vi "Reset.vi"(8 "error in (no error)":errorcluster, 10 "gRPCid":T4, 11 "ctet_dmm":T1) -> (0 "error out":errorcluster, 3 "ctet_dmm out":T1)   [LabVIEW 2019, in "ctet_dmm User Library.lvlib"]
uses:
  ctet_dmm User Library.lvlib
  Servers/ctet_dmm/gRPC lvSupport/Server API/typeDefs/grpcId.ctl
  Types/ctet_dmm.ctl
  Servers/ctet_dmm/ctet_dmm Class/RPC Messages/measurementservice_DMMConfigResponse/measurementservice_DMMConfigResponse_Data.ctl
  Servers/ctet_dmm/ctet_dmm Class/RPC Messages/measurementservice_ErrorOut/measurementservice_ErrorOut_Data.ctl
  Servers/ctet_dmm/ctet_dmm Class/RPC Messages/measurementservice_DMMResetResponse/measurementservice_DMMResetResponse_Data.ctl
  Servers/ctet_dmm/ctet_dmm Class/ctet_dmm.lvclass
  Servers/ctet_dmm/gRPC lvSupport/gprc-lvsupport.lvlib
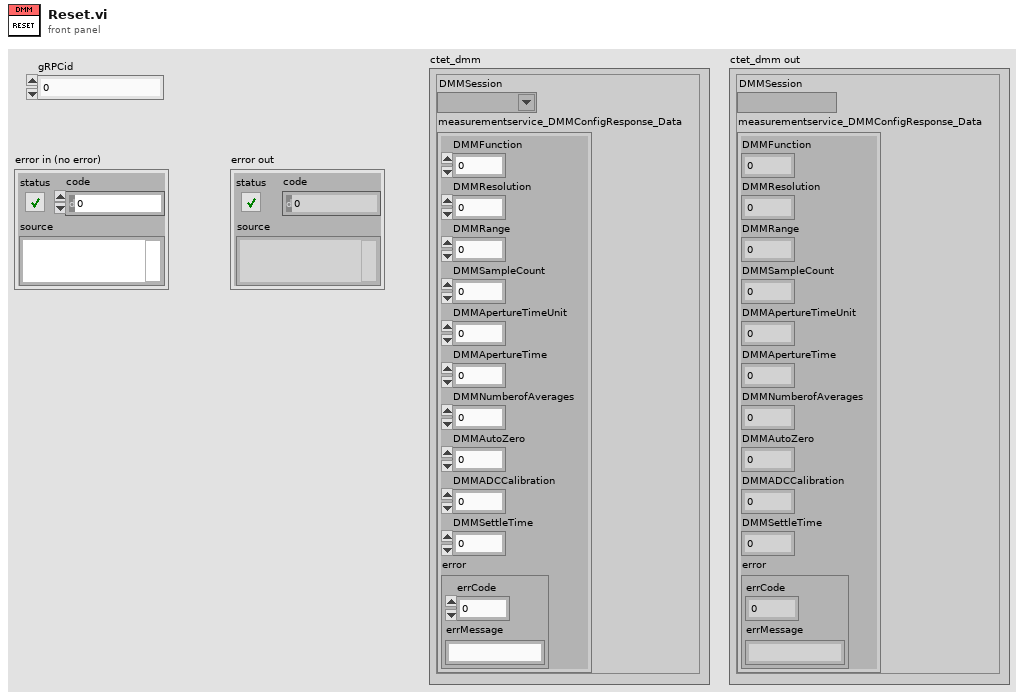
[diagram p1: front panel]
types:
  T1 = typedef "ctet_dmm User Library.lvlib/ctet_dmm.ctl" = cluster{"DMMSession":refnum<k15>, "measurementservice_DMMConfigResponse_Data":T2}
  T2 = typedef "ctet_dmm.lvlib/ctet_dmm.lvclass/measurementservice_DMMConfigResponse_Data.ctl" = cluster{"DMMFunction":i64, "DMMResolution":dbl, "DMMRange":dbl, "DMMSampleCount":i64, "DMMApertureTimeUnit":i64, "DMMApertureTime":dbl, "DMMNumberofAverages":i64, "DMMAutoZero":i64, "DMMADCCalibration":i64, "DMMSettleTime":dbl, "error":T3}
  T3 = typedef "ctet_dmm.lvlib/ctet_dmm.lvclass/measurementservice_ErrorOut_Data.ctl" = cluster{"errCode":i64, "errMessage":string}
  T4 = typedef "ctet_dmm.lvlib/gprc-lvsupport.lvlib/grpcId.ctl" = u64
  T5 = typedef "ctet_dmm.lvlib/ctet_dmm.lvclass/measurementservice_DMMResetResponse_Data.ctl" = cluster{"error":T3}
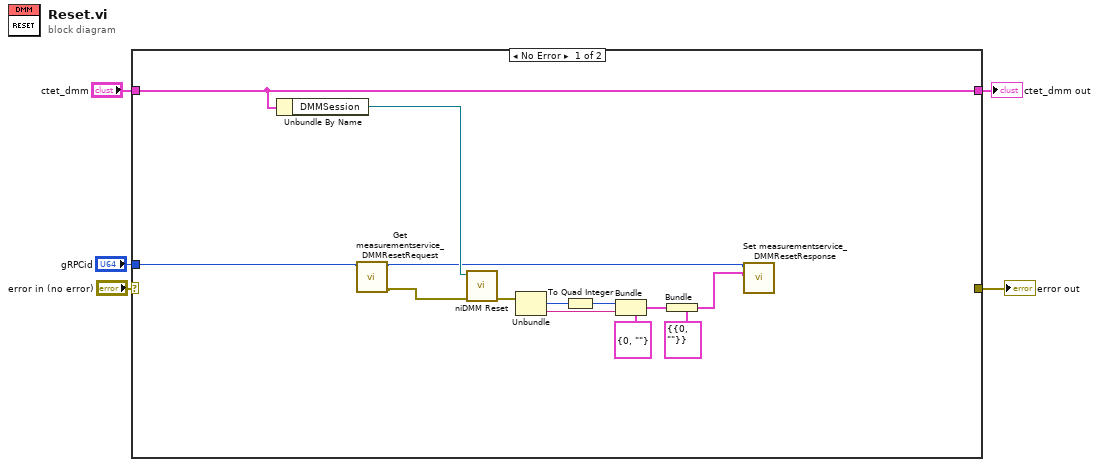
[diagram p0: block diagram]
diagram:
  n1 = case shown="No Error" "error in (no error)" {
    selector: "error in (no error)" -> [_ w20]
    tunnel: [_ w20] -> w5
    tunnel: "gRPCid" -> [w12 _]
    tunnel: "ctet_dmm" -> [w13 w19]
    tunnel: [w13 w19] -> w1
    frame No Error {
      n2 = Unbundle By Name(w13) -> ("DMMSession"=w14:refnum<k15>)
      n3 = call "Get measurementservice_DMMResetRequest.vi"("gRPCid"=w12) -> ("error out"=w11:errorcluster, "gRPCid out"=w10:T4)  [unwired: 8 in, 1 out]
      n4 = call <instrlib>:"niDMM Reset.vi"("error in (no error)"=w11, "instrument handle"=w14) -> ("error out"=w18:errorcluster)  [unwired: 8 in, 1 out]
      n5 = Unbundle(w18) -> ("code"=w16:i32, "source"=w17:string)  [unwired: 1 out]
      n6 = To Quad Integer(1:w16) -> (0:w15:i64)
      n7 = Bundle(cluster=T3 {"errCode"=0, "errMessage"=""} ("error"), "errCode"=w15, "errMessage"=w17) -> (w6:T3)
      n8 = Bundle(cluster=T5 {"error"={"errCode"=0, "errMessage"=""}} ("measurementservice_DMMResetResponse_Data"), "error"=w6) -> (w9:T5)
      n9 = call "Set measurementservice_DMMResetResponse.vi"("Message Data"=w9, "gRPCid"=w10) -> ()  [unwired: 9 in, 1 out]
    }
    frame Error {
    }
  }
  "error out" <- w5
  "ctet_dmm out" <- w1
